vi "millisecond Time Check.vi"(11 "error in (no error)":errorcluster) -> (3 "error out":errorcluster, 5 "millisecond timer value":u32)   [LabVIEW 2020]
doc: "Returns system millisecond count. Error handling for flow control."
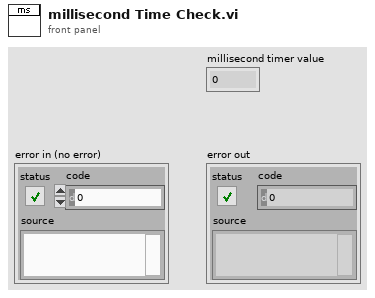
[diagram p1: front panel]
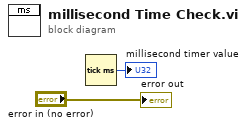
[diagram p0: block diagram]
diagram:
  n1 = Tick Count (ms)() -> (millisecond timer value=→"millisecond timer value":u32)
  "error out" <- "error in (no error)"
